vi "Dkm To Dmi.vi"(8 "error in (no error)":errorcluster, 11 "dKilo":dbl) -> (0 "error out":errorcluster, 3 "dmiles":dbl)   [LabVIEW 2023, in "POSCONV.lvlib"]
doc: "Converts double kilometres to double miles (One mile is 1.609344km)...\n\n\n\n\n\ndouble DkmToDmi(double dKilo);"
uses:
  POSCONV.lvlib
  C:/Users/J Gordon/Documents/Rail Tech/TV-HR/02 - Code/Modules/POSCONV/POSCONV.dll
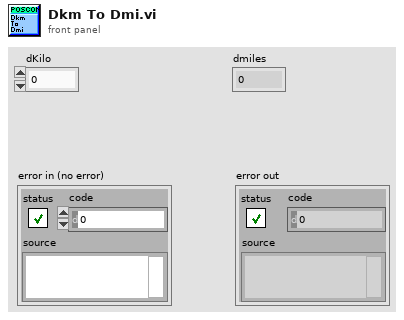
[diagram p1: front panel]
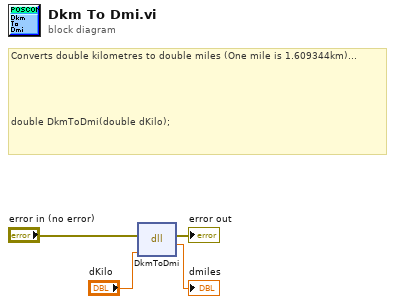
[diagram p0: block diagram]
diagram:
  # "Converts double kilometres to double miles (One mile is 1.609344km)...\n\n\n\n\n\ndouble DkmToDmi(double dKilo);"
  n1 = dll-call lib="C:/Users/J Gordon/Documents/Rail Tech/TV-HR/02 - Code/Modules/POSCONV/POSCONV.*" fn="DkmToDmi"(error in="error in (no error)", "dKilo"="dKilo") -> (error out=→"error out":errorcluster, →"dmiles":dbl)  [unwired: 3 in, 1 out]
